vi "PING网络状态.vi"() -> ()   [LabVIEW 2016, in "环境动力监测库.lvlib"]
uses:
  <vilib>/ptbypt/NI_PtbyPt.lvlib
panel:
  out "网络状态":bool
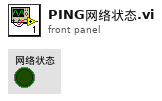
[diagram p1: front panel]
types:
  T1 = cluster{"网络参数":cluster{"网络状态":bool, "本机IP":string[]}, "电源管理":cluster{"电源管理":bool, "氨氮电源":bool, "总磷电源":bool, "总氮电源":bool, "多参数电源":bool, "CODMn电源":bool, "CODCr电源":bool, "灯带电源":bool, "照明电源":bool}, "北斗-GPS":cluster{"GPS":cluster{"经度:":sgl, "纬度: ":sgl, "GPS监测":bool}, "北斗":cluster{"经度:":sgl, "纬度:":sgl, "北斗监测":bool}}}
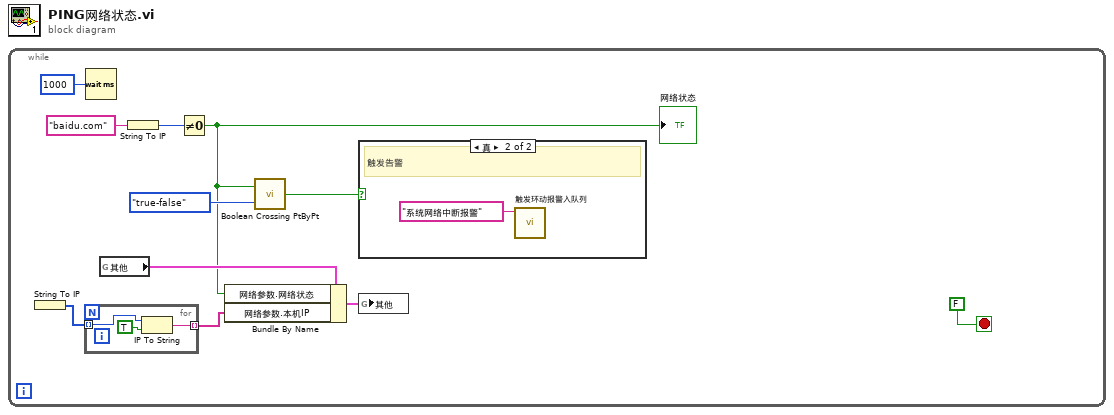
[diagram p0: block diagram]
diagram:
  n1 = while {
    stop <- FALSE stop-if-true
    n2 = String To IP() -> (0:w2:u32[])  [unwired: 1 in]
    n3 = for {
      tunnel: w2 -> [w13] mode=indexing
      tunnel: [w12] -> w1 mode=indexing
      n4 = IP To String(1:TRUE ("句点符号？(F)"), 2:w13) -> (0:w12:string)
    }
    n5 = Wait (ms)(milliseconds to wait=u32 1000 ("等待时间（毫秒）")) -> ()  [unwired: 1 out]
    n6 = global read "内部交互全局变量.vi" "其他"() -> (w6:T1)
    n7 = String To IP(1:"baidu.com" ("地址")) -> (0:w10:u32)
    n8 = Not Equal To 0?(x=w10) -> (x != 0?=w3:bool)
    "网络状态" <- w3
    n9 = Bundle By Name(cluster=w6, "网络参数.网络状态"=w3, "网络参数.本机IP"=w1) -> (w7:T1)
    n10 = call <vilib>:"Boolean Crossing PtByPt.vi"("direction"=enum16{"either", "false-true", "true-false"}."true-false", "input"=w3) -> ("crossing"=w4:bool)  [unwired: 1 in]
    n11 = case shown="真" w4 {
      frame False {
      }
      frame True {
        # "触发告警"
        n12 = call "触发环动报警入队列.vi"("报警内容"="系统网络中断报警") -> ()  [unwired: 11 in]
      }
    }
    n13 = global write "内部交互全局变量.vi" "其他"(w7) -> ()
  }
